vi "Drag Over.vi"(8 "error in (no error)":errorcluster, 9 "Coords":T1, 10 "BetterDropOp":refnum<class "BetterDropOp.lvclass">, 11 "BetterHandle in":refnum<class "BetterHandle.lvclass">) -> (0 "error out":errorcluster, 2 "Drag Accepted?":bool, 3 "BetterHandle out":refnum<class "BetterHandle.lvclass">)   [LabVIEW 2020, in "BetterDragAndDrop.lvlib" / "BetterHandle.lvclass"]
uses:
  BetterHandle.lvclass
  BetterDropOp/BetterDropOp.lvclass
  <vilib>/Utility/miscctls.llb/LVPoint32TypeDef.ctl
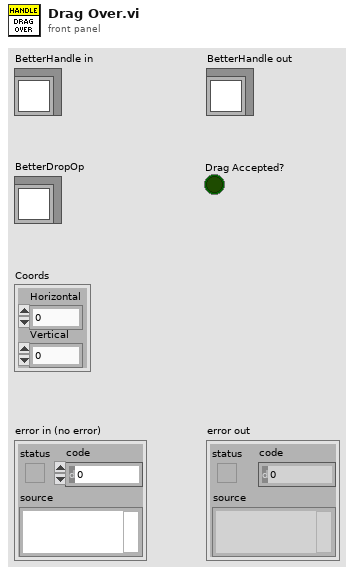
[diagram p1: front panel]
types:
  T1 = typedef "LVPoint32TypeDef.ctl" = cluster{"Horizontal":i32, "Vertical":i32}
  T2 = typedef "BetterDragAndDrop.lvlib/BetterHandle.lvclass/DragOver Output.ctl" = cluster{"Displayed Row":i32, "Position":T3, "Row's TreeItem index":i32, "indent":i32, "Accepted?":bool, "Insertion index":i32, "Top left visible TreeItem index":i32, "Bar type":T4}
  T3 = typedef "BetterDragAndDrop.lvlib/BetterHandle.lvclass/DragOverPosition.ctl" = enum16{"On Row", "Inbetween"}
  T4 = typedef "BetterDragAndDrop.lvlib/BetterHorizontalBar.lvclass/Horizontal Bar Enumeration.ctl" = enum16{"None", "only bar", "tilda up"}
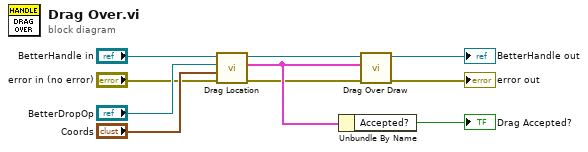
[diagram p0: block diagram]
diagram:
  n1 = call-dynamic "Drag Location.vi"("error in (no error)"="error in (no error)", "Coords"="Coords", "BetterDropOp"="BetterDropOp", "BetterHandle in"="BetterHandle in") -> ("error out"=w2:errorcluster, "DragOver Output"=w3:T2, "BetterHandle out"=w5:refnum<class "BetterHandle.lvclass">)  [unwired: 5 in]
  n2 = Unbundle By Name(w3) -> ("Accepted?"=→"Drag Accepted?":bool)
  n3 = call-dynamic "Drag Over Draw.vi"("error in (no error)"=w2, "DragOver Output"=w3, "BetterHandle in"=w5) -> ("error out"=→"error out":errorcluster, "BetterHandle out"=→"BetterHandle out":refnum<class "BetterHandle.lvclass">)  [unwired: 7 in]
